vi "Modify DG.vi"(7 "Settings":T1={"T Delay (µs)"=0.0, "T Set Back"=1.0, "T Triggers"=1, "T Active"=TRUE, "T Polarity"=TRUE, "T Term"=TRUE, "T Drive"=FALSE, "A Delay (µs)"=1.0, "A Set Back"=3.0, "A Triggers"=1, "A Active"=TRUE, "A Polarity"=TRUE, "A Term"=TRUE, "A Drive"=FALSE, "B Delay (µs)"=2.0, "B Set Back"=4.0, "B Triggers"=1, "B Active"=TRUE, "B Polarity"=TRUE, "B Term"=TRUE, "B Drive"=FALSE, "Gate A*B"=FALSE, "Output\nLevel"=1, "Trigger\nTerminate"=TRUE, "Clock\nEnable"=TRUE, "Internal\nClock (µs)"=10000.0, "Trigger\nLevel"=1.0, "Stop\nTrigger"=10, "Ocillator\nDivide By"=1, "Clock Source"=1, "Gate Divider"=1, "Positive\nGate"=FALSE, "Trigger\nSource"=TRUE, "Internal\nArming"=FALSE, "Software\nTrigger"=FALSE, "Trigger\nSlope"=TRUE, "Stop on\nPreset"=FALSE, "Trigger\nOperation"=TRUE, "Trigger\nEnable"=TRUE} {"B Set Back" min=0.0 format="%.3f"; "A Set Back" min=0.0 format="%.3f"; "T Set Back" min=0.0 format="%.3f"; "Clock Source" items=["Internal Oscillator"=1, "External Trigger"=2, "Trigger & Oscillator"=3, "Master Slave Bus"=4]; "Trigger\nLevel" min=0.0 format="%.3f"; "Output\nLevel" items=["TTL"=1, "NIM"=2, "ECL"=3]; "Internal\nClock (µs)" min=0.0 format="%.4f"; "B Delay (µs)" min=0.0 format="%.3f"; "A Delay (µs)" min=0.0 format="%.3f"; "T Delay (µs)" min=0.0 format="%.3f"}, 8 "error in (no error)":errorcluster, 11 "DG Number":i32) -> (0 "error out":errorcluster)   [LabVIEW 2009, in "POLARIS BME DG.lvlib"]
doc: "unsigned long Modify_DG(unsigned long OutputModulo_T0, BOOL Active_T0, BOOL Positive_T0, BOOL Terminate_T0, BOOL HighDrive_T0, unsigned long OutputModulo_A, BOOL Active_A, BOOL Positive_A, BOOL Terminate_A, BOOL HighDrive_A, unsigned long OutputModulo_B, BOOL Active_B, BOOL Positive_B, BOOL Terminate_B, BOOL HighDrive_B, unsigned long OutputLevel, BOOL TriggerTerminate, BOOL ClockEnable, unsigned long PresetValue, unsigned long ClockSource, unsigned long GateDivider, BOOL PositiveGate, BOOL InternalTrigger, BOOL InternalArm, BOOL SoftwareTrigger, BOOL RisingEdge, BOOL StopOnPreset, BOOL ResetWhenDone, BOOL TriggerEnable, long DG_Number);"
uses:
  POLARIS BME DG.lvlib
  Settings.ctl
  BME DLL/DelayGenerator.dll
panel:
  # "NOTICE -- YOU MUST LEAVE THIS NOTICE IN PLACE.  PER THE TERMS OF THE LICENSE BELOW, YOU MAY SUBLICENSE THIS SOFTWARE \nIN ANY WAY THAT DOES NOT CONFLICT WITH THIS LICENSE.\n\n### BSD License (http://www.opensource.org/licenses/bsd-license.php) Begin ###\n \nCopyright (c) 2011, Applied Energetics, http://www.appliedenergetics.com,\n                               Richard Schwerdtfeger, <rschwerdtfeger@appliedenergetics.com>\n\nAll rights reserved.\n\nRedistribution and use in source and binary forms, with or without modification, are permitted provided that the \nfollowing conditions are met:\n\n    * Redistributions of source code must retain the above copyright notice, this list of conditions and the following disclaimer.\n    * Redistributions in binary form must reproduce the above copyright notice, this list of conditions and the following disclaimer \n       in the documentation and/or other materials provided with the distribution.\n    * Neither the name of Richard Schwerdtfeger, Applied Energetics, Inc., nor the names of its contributors may be used to \n       endorse or promote products derived from this software without specific prior written permission.\n\nTHIS SOFTWARE IS PROVIDED BY THE COPYRIGHT HOLDERS AND CONTRIBUTORS \"AS IS\" AND ANY EXPRESS OR IMPLIED WARRANTIES, \nINCLUDING, BUT NOT LIMITED TO, THE IMPLIED WARRANTIES OF MERCHANTABILITY AND FITNESS FOR A PARTICULAR PURPOSE ARE \nDISCLAIMED. IN NO EVENT SHALL THE COPYRIGHT OWNER OR CONTRIBUTORS BE LIABLE FOR ANY DIRECT, INDIRECT, INCIDENTAL,\n SPECIAL, EXEMPLARY, OR CONSEQUENTIAL DAMAGES (INCLUDING, BUT NOT LIMITED TO, PROCUREMENT OF SUBSTITUTE GOODS OR \nSERVICES; LOSS OF USE, DATA, OR PROFITS; OR BUSINESS INTERRUPTION) HOWEVER CAUSED AND ON ANY THEORY OF LIABILITY, \nWHETHER IN CONTRACT, STRICT LIABILITY, OR TORT (INCLUDING NEGLIGENCE OR OTHERWISE) ARISING IN ANY WAY OUT OF THE USE \nOF THIS SOFTWARE, EVEN IF ADVISED OF THE POSSIBILITY OF SUCH DAMAGE.\n\n### BSD License End ###"
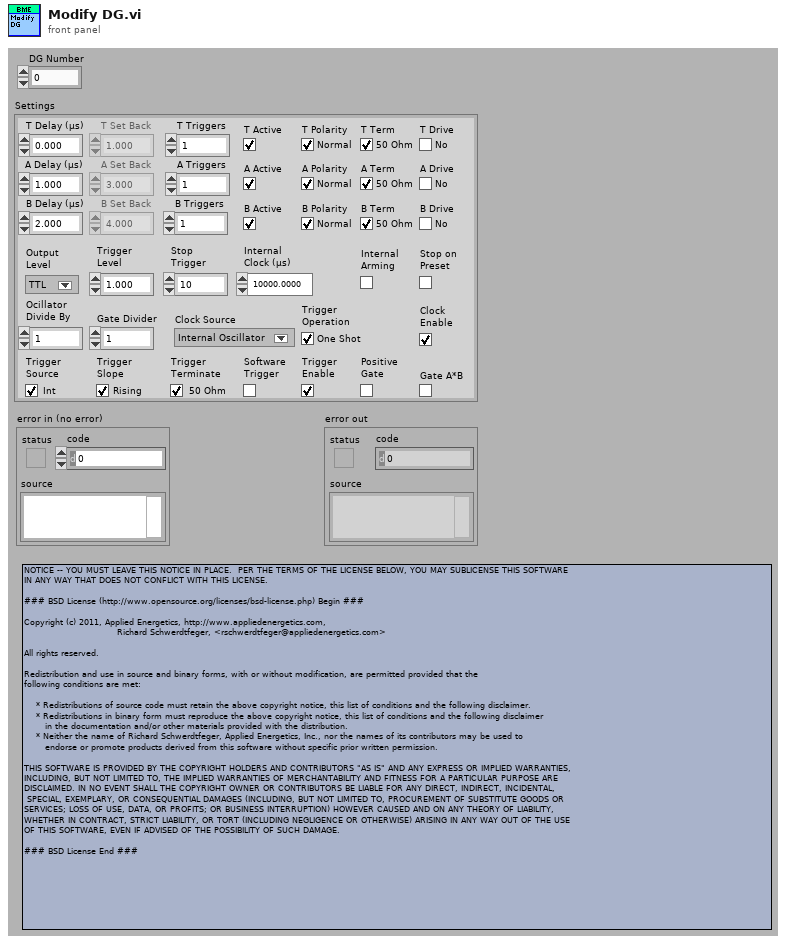
[diagram p1: front panel]
types:
  T1 = typedef "POLARIS BME DG.lvlib/Settings.ctl" = cluster{"T Delay (µs)":dbl, "T Set Back":dbl, "T Triggers":u16, "T Active":bool, "T Polarity":bool, "T Term":bool, "T Drive":bool, "A Delay (µs)":dbl, "A Set Back":dbl, "A Triggers":u16, "A Active":bool, "A Polarity":bool, "A Term":bool, "A Drive":bool, "B Delay (µs)":dbl, "B Set Back":dbl, "B Triggers":u16, "B Active":bool, "B Polarity":bool, "B Term":bool, "B Drive":bool, "Gate A*B":bool, "Output\nLevel":u32, "Trigger\nTerminate":bool, "Clock\nEnable":bool, "Internal\nClock (µs)":dbl, "Trigger\nLevel":dbl, "Stop\nTrigger":u32, "Ocillator\nDivide By":u16, "Clock Source":u32, "Gate Divider":u32, "Positive\nGate":bool, "Trigger\nSource":bool, "Internal\nArming":bool, "Software\nTrigger":bool, "Trigger\nSlope":bool, "Stop on\nPreset":bool, "Trigger\nOperation":bool, "Trigger\nEnable":bool}
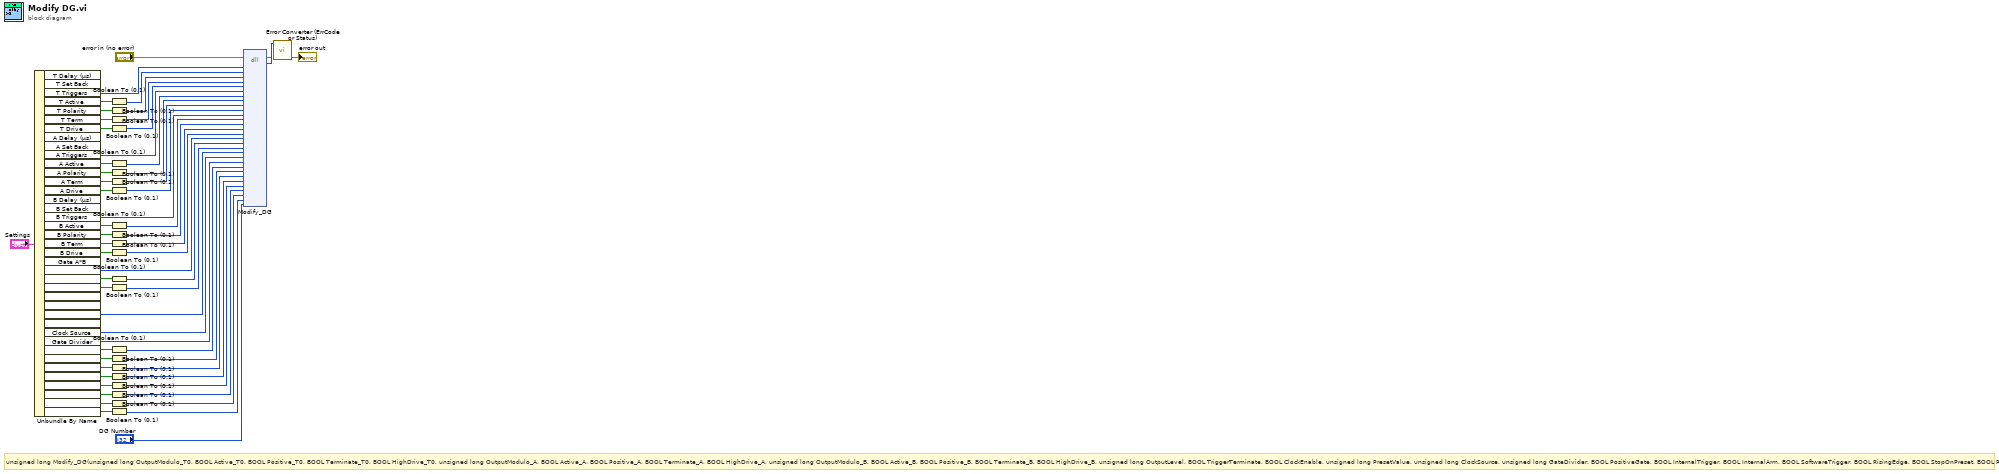
[diagram p0: block diagram]
diagram:
  # "unsigned long Modify_DG(unsigned long OutputModulo_T0, BOOL Active_T0, BOOL Positive_T0, BOOL Terminate_T0, BOOL HighDrive_T0, unsigned long OutputModulo_A, BOOL Active_A, BOOL Positive_A, BOOL Terminate_A, BOOL HighDrive_A, unsigned long OutputModulo_B, BOOL Active_B, BOOL Positive_B, BOOL Terminate_B, BOOL HighDrive_B, unsigned long OutputLevel, BOOL TriggerTerminate, BOOL ClockEnable, unsigned long PresetValue, unsigned long ClockSource, unsigned long GateDivider, BOOL PositiveGate, BOOL InternalTrigger, BOOL InternalArm, BOOL SoftwareTrigger, BOOL RisingEdge, BOOL StopOnPreset, BOOL ResetWhenDone, BOOL TriggerEnable, long DG_Number);"
  n1 = Unbundle By Name("Settings") -> ("T Triggers"=w3:u16, "T Active"=w30:bool, "T Polarity"=w31:bool, "T Term"=w51:bool, "T Drive"=w50:bool, "A Triggers"=w2:u16, "A Active"=w32:bool, "A Polarity"=w49:bool, "A Term"=w33:bool, "A Drive"=w34:bool, "B Triggers"=w1:u16, "B Active"=w35:bool, "B Polarity"=w36:bool, "B Term"=w37:bool, "B Drive"=w38:bool, "Output\nLevel"=w17:u32, "Trigger\nTerminate"=w39:bool, "Clock\nEnable"=w40:bool, "Stop\nTrigger"=w14:u32, "Clock Source"=w13:u32, "Gate Divider"=w12:u32, "Positive\nGate"=w41:bool, "Trigger\nSource"=w42:bool, "Internal\nArming"=w43:bool, "Software\nTrigger"=w44:bool, "Trigger\nSlope"=w45:bool, "Stop on\nPreset"=w46:bool, "Trigger\nOperation"=w47:bool, "Trigger\nEnable"=w48:bool)  [unwired: 10 out]
  n2 = Boolean To (0,1)(Boolean=w30) -> (0, 1=w29:i16)
  n3 = Boolean To (0,1)(Boolean=w31) -> (0, 1=w28:i16)
  n4 = Boolean To (0,1)(Boolean=w51) -> (0, 1=w27:i16)
  n5 = Boolean To (0,1)(Boolean=w50) -> (0, 1=w26:i16)
  n6 = Boolean To (0,1)(Boolean=w32) -> (0, 1=w25:i16)
  n7 = Boolean To (0,1)(Boolean=w49) -> (0, 1=w24:i16)
  n8 = Boolean To (0,1)(Boolean=w33) -> (0, 1=w23:i16)
  n9 = Boolean To (0,1)(Boolean=w34) -> (0, 1=w22:i16)
  n10 = Boolean To (0,1)(Boolean=w35) -> (0, 1=w21:i16)
  n11 = Boolean To (0,1)(Boolean=w36) -> (0, 1=w20:i16)
  n12 = Boolean To (0,1)(Boolean=w37) -> (0, 1=w19:i16)
  n13 = Boolean To (0,1)(Boolean=w38) -> (0, 1=w18:i16)
  n14 = Boolean To (0,1)(Boolean=w39) -> (0, 1=w16:i16)
  n15 = Boolean To (0,1)(Boolean=w40) -> (0, 1=w15:i16)
  n16 = Boolean To (0,1)(Boolean=w41) -> (0, 1=w11:i16)
  n17 = Boolean To (0,1)(Boolean=w42) -> (0, 1=w10:i16)
  n18 = Boolean To (0,1)(Boolean=w43) -> (0, 1=w9:i16)
  n19 = Boolean To (0,1)(Boolean=w44) -> (0, 1=w8:i16)
  n20 = Boolean To (0,1)(Boolean=w45) -> (0, 1=w7:i16)
  n21 = Boolean To (0,1)(Boolean=w46) -> (0, 1=w6:i16)
  n22 = Boolean To (0,1)(Boolean=w47) -> (0, 1=w5:i16)
  n23 = Boolean To (0,1)(Boolean=w48) -> (0, 1=w4:i16)
  n24 = dll-call lib="C:/CS Framework/LVSCC/LV2009/GPL/Projects/cs-framework/CSClass/CSPOLARIS/POLARIS BME DG/BME DLL/DelayGenerator.*" fn="Modify_DG"(error in="error in (no error)", "OutputModulo_T0"=w3, "Active_T0"=w29, "Positive_T0"=w28, "Terminate_T0"=w27, "HighDrive_T0"=w26, "OutputModulo_A"=w2, "Active_A"=w25, "Positive_A"=w24, "Terminate_A"=w23, "HighDrive_A"=w22, "OutputModulo_B"=w1, "Active_B"=w21, "Positive_B"=w20, "Terminate_B"=w19, "HighDrive_B"=w18, "OutputLevel"=w17, "TriggerTerminate"=w16, "ClockEnable"=w15, "PresetValue"=w14, "ClockSource"=w13, "GateDivider"=w12, "PositiveGate"=w11, "InternalTrigger"=w10, "InternalArm"=w9, "SoftwareTrigger"=w8, "RisingEdge"=w7, "StopOnPreset"=w6, "ResetWhenDone"=w5, "TriggerEnable"=w4, "DG_Number"="DG Number") -> (error out=w54:errorcluster, w57:u32)  [unwired: 7 in, 26 out]
  n25 = call "Error Converter (ErrCode or Status).vi"("error in (no error)"=w54, "error code"=w57) -> ("error out"=→"error out":errorcluster)  [unwired: 9 out]
